vi "VI Server_M_ClmnListBox_1orMoreSelection_ItemNames_GET.vi"(7 "Label":string, 8 "error in":errorcluster, 10 "SingleInstance":bool=TRUE, 11 "VI Server.RefsCluster":T2) -> (0 "error out":errorcluster, 1 "Multicolumn Listbox.Ref":refnum<vi>, 2 "Item Names":string[][](array[string]), 3 "VI Server.RefsCluster.DUP":T2, 4 "Selected Cell":T1, 5 "Item Symbols":i32[](array[numeric]), 6 "Value":i32[](array[numeric]))   [LabVIEW 2020]
uses:
  VI Server_TypeDefs/VI Server_RefsCluster.ctl
  <vilib>/Utility/miscctls.llb/LVRowAndColumnTypeDef.ctl
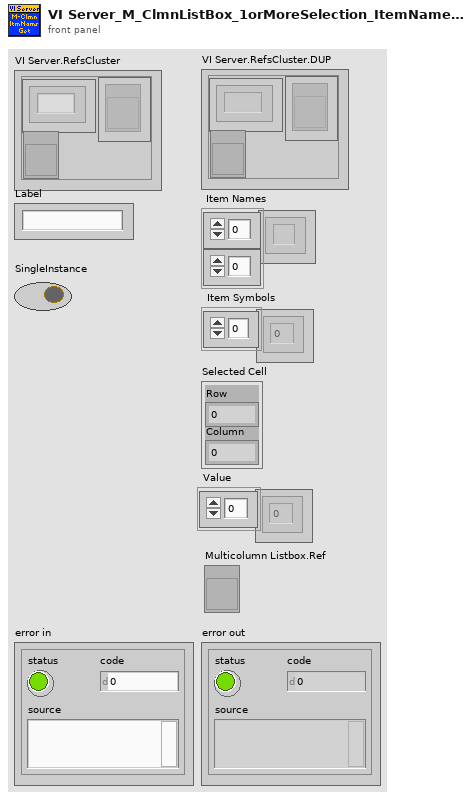
[diagram p1: front panel]
types:
  T1 = typedef "LVRowAndColumnTypeDef.ctl" = cluster{"Row":i32, "Column":i32}
  T2 = typedef "VI Server_RefsCluster.ctl" = cluster{"Labels":string[], "Refs":refnum<vi>[], "VI Ref":refnum<vi>}
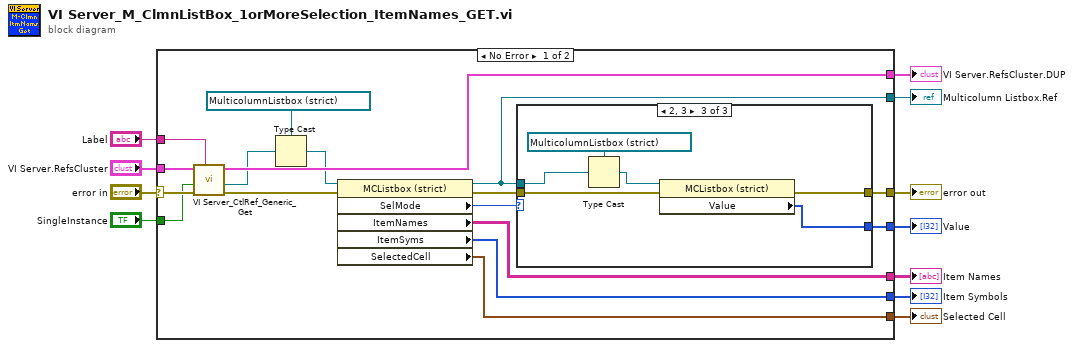
[diagram p0: block diagram]
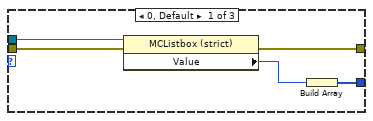
[diagram p2: hidden frame]
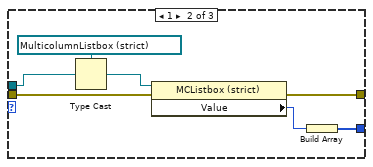
[diagram p3: hidden frame]
diagram:
  n1 = case shown="No Error" "error in" {
    selector: "error in" -> [w28 w48]
    tunnel: [w15 w48] -> w10
    tunnel: "VI Server.RefsCluster" -> [w27 w47]
    tunnel: [w26 w47] -> w8
    tunnel: "Label" -> [w25 _]
    tunnel: "SingleInstance" -> [w21 _]
    tunnel: [w20 _] -> w5
    tunnel: [w19 _] -> w4
    tunnel: [w17 _] -> w3
    tunnel: [w13 _] -> w2
    tunnel: [w12 _] -> w1
    frame No Error {
      n2 = call "VI Server_CtlRef_Generic_Get.vi"("Control.Label"=w25, "error in"=w28, "SingleInstance"=w21, "VI Server.RefsCluster"=w27) -> ("error out"=w23:errorcluster, "Control.Ref.Generic"=w24:refnum<vi>, "VI Server.RefsCluster.DUP"=w26:T2)  [unwired: 5 in]
      n3 = Type Cast(type=refnum<vi> refnum ("Multicolumn Listbox"), x=w24) -> (*(type *) &x=w22:refnum<vi>)
      n4 = property class="MCListbox (strict)"(reference=w22, error in=w23) -> (reference out=w12:refnum<vi>, error out=w16:errorcluster, "SelMode"=w14:i32, "ItemNames"=w17:string[][], "ItemSyms"=w19:i32[], "SelectedCell"=w20:T1)
      n5 = case shown="2, 3" w14 {
        tunnel: w16 -> [w33 w40 w46]
        tunnel: [w32 w39 w45] -> w15
        tunnel: w12 -> [w31 w35 w42]
        tunnel: [w29 w37 w44] -> w13
        frame 0, Default {
          n6 = property class="MCListbox (strict)"(reference=w31, error in=w33) -> (error out=w32:errorcluster, "Value"=w30:i32)  [unwired: 1 out]
          n7 = Build Array(w30) -> (w29:i32[])
        }
        frame 1 {
          n8 = Type Cast(type=refnum<vi> refnum ("Multicolumn Listbox"), x=w35) -> (*(type *) &x=w36:refnum<vi>)
          n9 = property class="MCListbox (strict)"(reference=w36, error in=w40) -> (error out=w39:errorcluster, "Value"=w38:i32)  [unwired: 1 out]
          n10 = Build Array(w38) -> (w37:i32[])
        }
        frame 2, 3 {
          n11 = Type Cast(type=refnum<vi> refnum ("Multicolumn Listbox"), x=w42) -> (*(type *) &x=w43:refnum<vi>)
          n12 = property class="MCListbox (strict)"(reference=w43, error in=w46) -> (error out=w45:errorcluster, "Value"=w44:i32[])  [unwired: 1 out]
        }
      }
    }
    frame Error {
    }
  }
  "VI Server.RefsCluster.DUP" <- w8
  "error out" <- w10
  "Value" <- w2
  "Selected Cell" <- w5
  "Item Symbols" <- w4
  "Item Names" <- w3
  "Multicolumn Listbox.Ref" <- w1
